vi "Create Dataset 3D Integer.vi"(4 "Size of dimension 2":u64, 6 "Size of dimension 1":u64, 8 "Chunk Sizes":u64[](array[numeric]), 9 "Dataset name":string, 10 "loc_id":i32, 11 "error in (no error)":errorcluster) -> (0 "Error code":i32, 2 "dataset_id":i32, 3 "error out":errorcluster)   [LabVIEW 2010]
uses:
  Release/HDF5Tools.dll
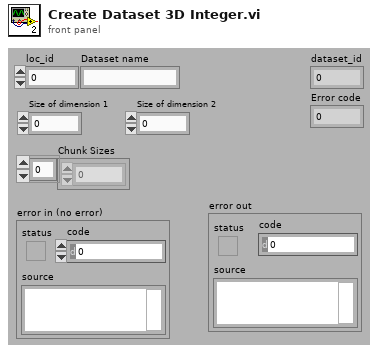
[diagram p1: front panel]
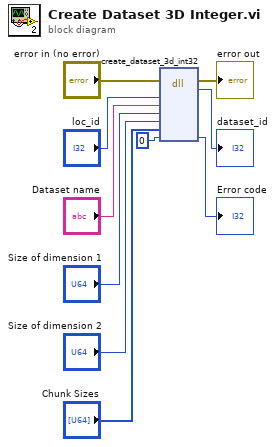
[diagram p0: block diagram]
diagram:
  n1 = dll-call lib="Z:/users/alex/projects/HDF5Tools/Release/HDF5Tools.dll" fn="create_dataset_3d_int32"(error in="error in (no error)", "loc_id"="loc_id", "name"="Dataset name", "dim1"="Size of dimension 1", "dim2"="Size of dimension 2", "chunks"="Chunk Sizes", "error"=0) -> (error out=→"error out":errorcluster, "dataset_id"=→"dataset_id":i32, "error"=→"Error code":i32)  [unwired: 7 in, 1 out]
